vi "Set_API_ID.vi"(8 "New API ID":i32, 9 "Index":i32, 10 "API Function Array In":cluster{string, "VI Reference":refnum<vi>}[](array[cluster]), 11 "Input Sequence":cluster{string, string[], dbl[], dbl}[](array[cluster])) -> (2 "API Function Array Out":cluster{string, "VI Reference":refnum<vi>}[](array[cluster]), 3 "Output Sequence":cluster{string, string[], dbl[], dbl}[](array[cluster]))   [LabVIEW 2011]
doc: "This VI allows the user to alter a command's API ID while still retaining its correlation with the appropriate polymorphic API VI reference."
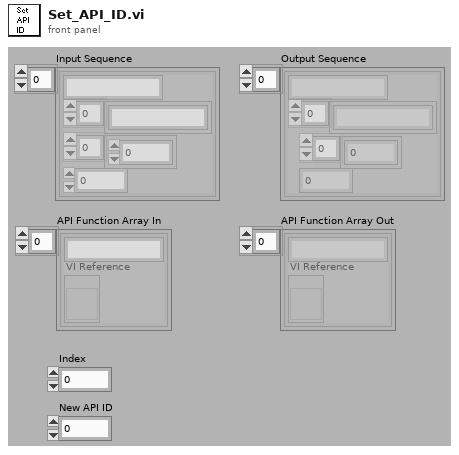
[diagram p1: front panel]
types:
  T1 = cluster{"String":string, "VI Reference":refnum<vi>}
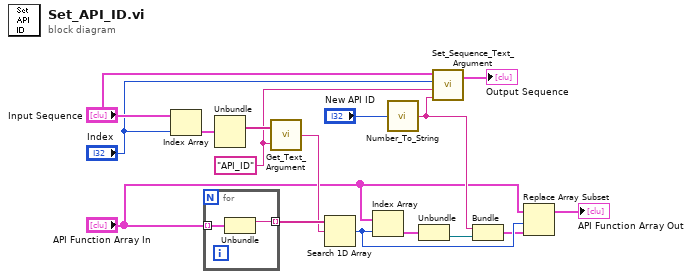
[diagram p0: block diagram]
diagram:
  w8 = "API_ID" ("Argument")
  n1 = Index Array(array="Input Sequence", index="Index") -> (element=w16:cluster{string, string[], dbl[], dbl})
  n2 = for {
    tunnel: "API Function Array In" -> [w18] mode=indexing
    tunnel: [w17] -> w14 mode=indexing
    n3 = Unbundle(w18) -> (w17:string)  [unwired: 1 out]
  }
  n4 = Unbundle(w16) -> (w15:string[])  [unwired: 3 out]
  n5 = call "Get_Text_Argument.vi"("Argument"=w8, "Argument List"=w15) -> ("Text"=w13:string)
  n6 = Search 1D Array(1D array=w14, element=w13) -> (index of element=w3:i32)  [unwired: 1 out]
  n7 = Index Array(array="API Function Array In", index=w3) -> (element=w12:cluster{string, "VI Reference":refnum<vi>})
  n8 = call "Number_To_String.vi"("Number"="New API ID") -> ("String"=w5:string)
  n9 = Unbundle(w12) -> ("VI Reference"=w11:refnum<vi>)  [unwired: 1 out]
  n10 = call "Set_Sequence_Text_Argument.vi"("Text"=w5, "Argument"=w8, "Index"="Index", "Input Sequence"="Input Sequence") -> ("Output Sequence"=→"Output Sequence":cluster{string, string[], dbl[], dbl}[])  [unwired: 1 out]
  n11 = Bundle("String"=w5, "VI Reference"=w11) -> (w2:T1)  [unwired: 1 out]
  n12 = Replace Array Subset(array="API Function Array In", new element=w2, index=w3) -> (→"API Function Array Out":cluster{string, "VI Reference":refnum<vi>}[])
